vi "02地址状态值.vi"(11 "unsigned byte array":u8[](array[numeric])) -> (0 "E2初始化失败":bool, 3 "故障":bool)   [LabVIEW 2012]
panel:
  out "第一组传感器故障":bool
  out "第二组传感器故障":bool
  out "霍尔故障":bool
  out "AD故障":bool
  out "超时故障":bool
  out "温度故障":bool
  out "超速故障":bool
  out "过流故障":bool
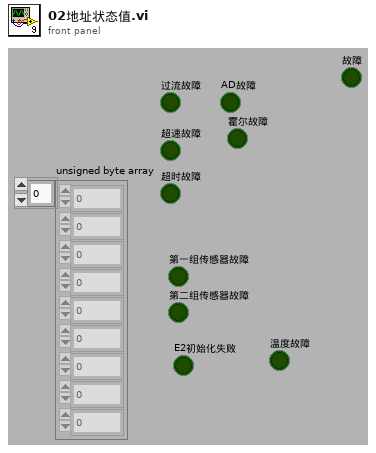
[diagram p1: front panel]
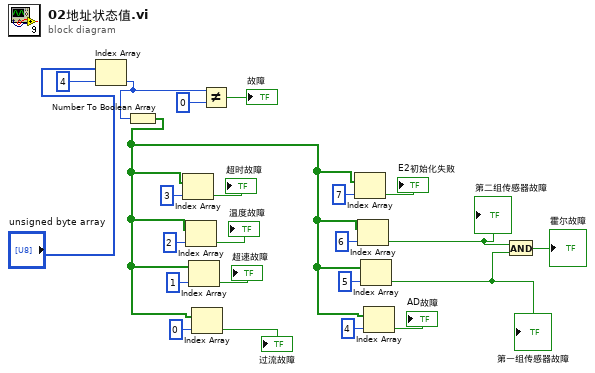
[diagram p0: block diagram]
diagram:
  n1 = Index Array(array="unsigned byte array", index=4 ("索引")) -> (element=w3:u8)
  n2 = Number To Boolean Array(number=w3) -> (Boolean array=w12:bool[])
  n3 = Index Array(array=w12, index=3 ("索引")) -> (element=→"超时故障":bool)
  n4 = Index Array(array=w12, index=2 ("索引")) -> (element=→"温度故障":bool)
  n5 = Index Array(array=w12, index=1 ("索引")) -> (element=→"超速故障":bool)
  n6 = Index Array(array=w12, index=0 ("索引")) -> (element=→"过流故障":bool)
  n7 = Not Equal?(x=w3, y=u8 0) -> (x != y?=→"故障":bool)
  n8 = Index Array(array=w12, index=7 ("索引")) -> (element=→"E2初始化失败":bool)
  n9 = Index Array(array=w12, index=6 ("索引")) -> (element=w19:bool)
  "第二组传感器故障" <- w19
  n10 = Index Array(array=w12, index=5 ("索引")) -> (element=w20:bool)
  "第一组传感器故障" <- w20
  n11 = Index Array(array=w12, index=4 ("索引")) -> (element=→"AD故障":bool)
  n12 = And(x=w19, y=w20) -> (x .and. y?=→"霍尔故障":bool)
